vi "1DBangBang.vi"(0 "object in":refnum<class "Navigation.lvclass">, 1 "Target":dbl, 2 "Position":dbl, 3 "curVel":dbl, 4 "destVel":dbl, 5 "error in (no error)":errorcluster, 8 "Stop":bool, 9 "acceleration":dbl=1.0, 13 "v_max":dbl format="%#_13g") -> (14 "object out":refnum<class "Navigation.lvclass">, 17 "outputVel":dbl, 19 "error out":errorcluster)   [LabVIEW 2023, in "Navigation.lvclass"]
uses:
  Navigation.lvclass
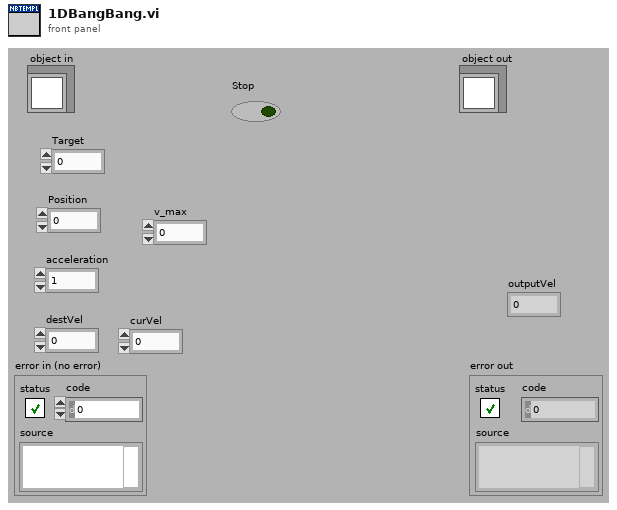
[diagram p1: front panel]
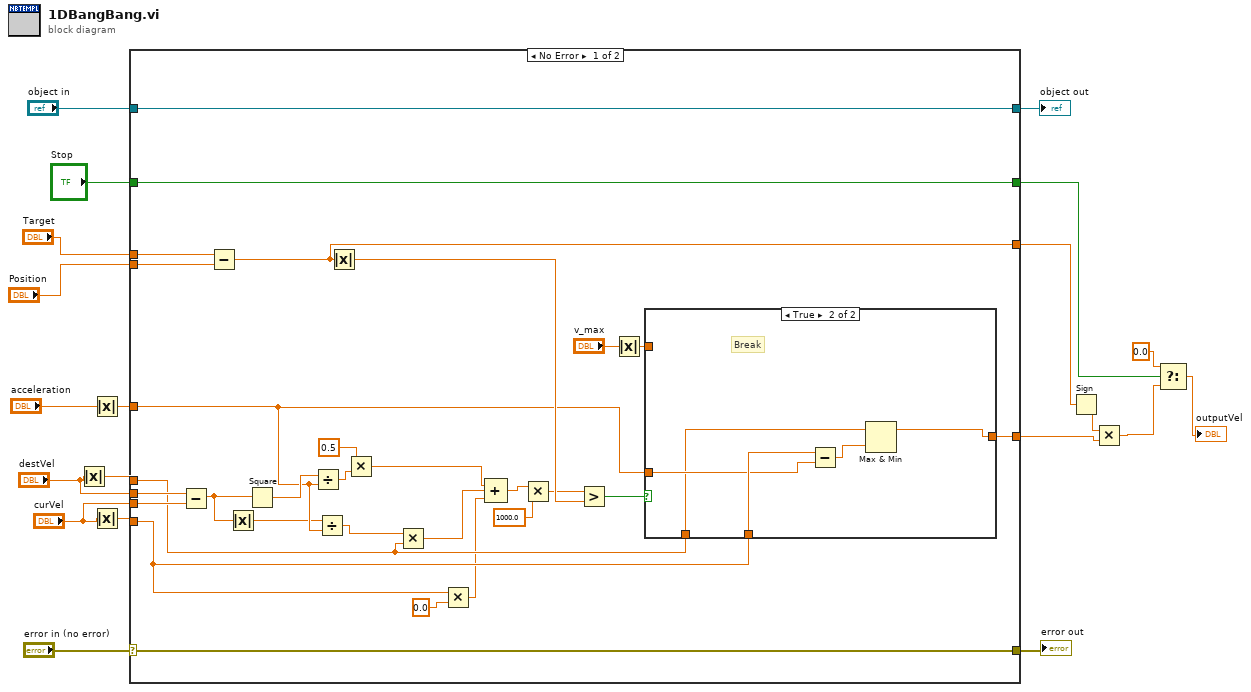
[diagram p0: block diagram]
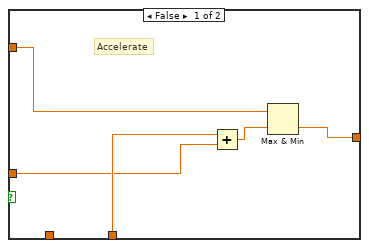
[diagram p2: hidden frame]
diagram:
  n1 = Absolute Value(x="destVel") -> (abs(x)=w11:dbl)
  n2 = Absolute Value(x="acceleration") -> (abs(x)=w12:dbl)
  n3 = Absolute Value(x="curVel") -> (abs(x)=w10:dbl)
  n4 = case shown="No Error" "error in (no error)" {
    selector: "error in (no error)" -> [w48 w61]
    tunnel: [w48 w61] -> w19
    tunnel: [w49 w60] -> w17
    tunnel: "object in" -> [w49 w60]
    tunnel: w11 -> [w28 _]
    tunnel: w10 -> [w25 _]
    tunnel: w12 -> [w38 _]
    tunnel: "Target" -> [w41 _]
    tunnel: "Position" -> [w40 _]
    tunnel: [w37 _] -> w7
    tunnel: "Stop" -> [w21 _]
    tunnel: [w34 _] -> w9
    tunnel: "destVel" -> [w30 _]
    tunnel: "curVel" -> [w29 _]
    tunnel: [w21 _] -> w4
    frame No Error {
      n5 = Subtract(x=w30, y=w29) -> (x-y=w27:dbl)
      n6 = Subtract(x=w41, y=w40) -> (x-y=w34:dbl)
      n7 = Absolute Value(x=w27) -> (abs(x)=w26:dbl)
      n8 = Square(x=w27) -> (x^2=w47:dbl)
      n9 = Divide(x=w47, y=w38) -> (x/y=w46:dbl)
      n10 = Divide(x=w26, y=w38) -> (x/y=w44:dbl)
      n11 = Absolute Value(x=w34) -> (abs(x)=w39:dbl)
      n12 = Multiply(x=0.5, y=w46) -> (x*y=w42:dbl)
      n13 = Multiply(x=w44, y=w28) -> (x*y=w43:dbl)
      n14 = Multiply(x=w25, y=0.0) -> (x*y=w23:dbl)
      n15 = Compound Arithmetic op=ADD(w42, w43, w23) -> (w33:dbl)
      n16 = Multiply(x=w33, y=1000.0) -> (x*y=w31:dbl)
      n17 = Greater?(x=w31, y=w39) -> (0:w22:bool)
      n18 = Absolute Value(x="v_max") -> (abs(x)=w35:dbl)
      n19 = case shown="True" w22 {
        tunnel: w28 -> [_ w56]
        tunnel: w25 -> [w53 w59]
        tunnel: w38 -> [w50 w57]
        tunnel: [w51 w55] -> w37
        tunnel: w35 -> [w52 _]
        frame False {
          # "Accelerate"
          n20 = Add(x=w53, y=w50) -> (x+y=w54:dbl)
          n21 = Max & Min(x=w52, y=w54) -> (min(x,y)=w51:dbl)  [unwired: 1 out]
        }
        frame True {
          # "Break"
          n22 = Subtract(x=w59, y=w57) -> (x-y=w58:dbl)
          n23 = Max & Min(x=w56, y=w58) -> (max(x,y)=w55:dbl)  [unwired: 1 out]
        }
      }
    }
    frame Error {
    }
  }
  "error out" <- w19
  "object out" <- w17
  n24 = Sign(1:w9) -> (0:w8:dbl)
  n25 = Multiply(x=w8, y=w7) -> (x*y=w3:dbl)
  n26 = Select(t=0.0, s=w4, f=w3) -> (s? t:f=→"outputVel":dbl)
